vi "Kinesis no front panel.vi"() -> ()   [LabVIEW 2017]
uses:
  D:/upwork/Laser Measurement Tool/Laser/tests/KIM101/Thorlabs.MotionControl.KCube.DCServoCLI.dll
  Thorlabs.MotionControl.KCube.DCServoCLI.dll
  D:/upwork/Laser Measurement Tool/Laser/tests/KIM101/Thorlabs.MotionControl.Controls.dll
  Thorlabs.MotionControl.Controls.dll
panel:
  in  "SerialNumber":string
  out "Control reference":refnum<k24>
  out "error out":errorcluster
  out "Device reference":refnum<k24>
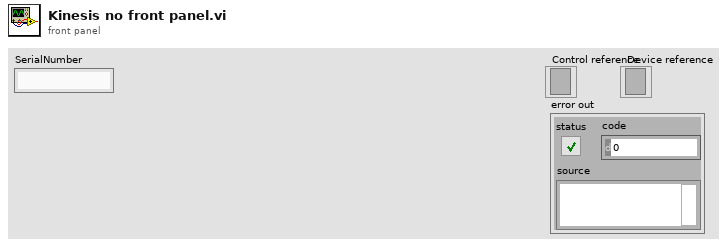
[diagram p1: front panel]
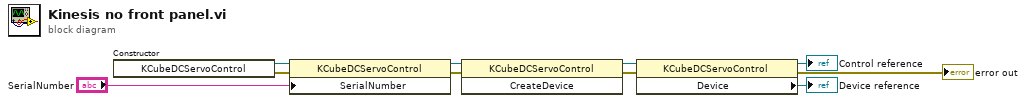
[diagram p0: block diagram]
diagram:
  n1 = constructor class="KCubeDCServoControl"() -> (reference out=w10:refnum<k24>, error out=w9:errorcluster)  [unwired: 3 in, 1 out]
  n2 = property class="KCubeDCServoControl"(reference=w10, error in=w9, "SerialNumber"="SerialNumber") -> (reference out=w8:refnum<k24>, error out=w7:errorcluster)
  n3 = invoke class="KCubeDCServoControl" method="CreateDevice"(reference=w8, error in=w7) -> (reference out=w6:refnum<k24>, error out=w5:errorcluster)  [unwired: 1 in, 1 out]
  n4 = property class="KCubeDCServoControl"(reference=w6, error in=w5) -> (reference out=→"Control reference":refnum<k24>, error out=→"error out":errorcluster, "Device"=→"Device reference":refnum<k24>)
